vi "07_1.vi"() -> ()   [LabVIEW 2018]
uses:
  <userlib>/_OpenG.lib/array/array.llb/Remove Duplicates from 1D Array (String)__ogtk.vi
panel:
  out "Contained by Number":i32
  out "Contained by":string[](array[string])
  in  "Input":string="light chartreuse bags contain 1 mirrored yellow bag, 2 vibrant violet bags.\ndotted silver bags contain 2 dotted orange bags, 3 bright fuchsia bags, 5 bright tomato bags, 3 faded turquoise bags.\nplaid indigo bags contain 1 pale violet bag, 4 mirrored violet bags.\nfaded turquoise bags contain 5 faded lavender bags.\nstriped yellow bags contain 5 vibrant black bags, 1 mirrored gold bag.\ndull tan bags contain 1 vibrant aqua bag.\nstriped brown bags contain 1 vibrant orange bag, 1 posh bronze bag, 4 dim purple bags.\nbright teal bags contain 3 muted cyan bags, 2 drab white bags, 1 drab gray bag.\nwavy tan bags contain 4 wavy tomato bags, 1 dim tan bag.\nlight lavender bags contain 1 dotted black bag, 1 wavy maroon bag, 5 pale white bags, 1 clear tan bag.\ndull orange bags contain 5 bright brown bags, 1 muted gold bag, 4 vibrant black bags, 4 posh bronze bags.\nposh cyan bags contain 2 mirrored tomato bags, 5 light salmon bags, 1 faded brown bag, 4 vibrant red bags.\ndark lavender bags contain 2 faded purple bags.\ndark white bags contain 5 muted green bags.\nstriped olive bags contain 1 muted chartreuse bag.\nbright crimson bags contain 3 drab salmon bags, 1 faded plum bag, 4 shiny brown bags, 5 pale orange bags.\ndark tomato bags contain 5 dim aqua bags.\nlight olive bags contain 2 drab blue bags, 1 plaid purple bag.\nmuted gray bags contain 1 mirrored plum bag.\nbright salmon bags contain 3 striped plum bags, 1 dull silver bag, 4 striped indigo bags, 4 striped cyan bags.\nwavy gold bags contain 3 drab tomato bags, 5 pale gold bags, 1 plaid tan bag, 5 vibrant gold bags.\nmuted fuchsia bags contain 3 vibrant plum bags, 1 clear chartreuse bag, 1 pale white bag.\nlight purple bags contain 5 vibrant olive bags, 4 bright maroon bags, 3 posh tomato bags.\nvibrant gray bags contain 5 shiny silver bags.\nvibrant beige bags contain 2 pale crimson bags, 5 pale olive bags, 4 posh yellow bags, 3 dotted orange bags.\ndrab beige bags contain 3 faded gold bags, 5 mirrored fuchsia bags.\nlight white bags contain 1 vibrant fuchsia bag, 3 posh tomato bags, 4 muted chartreuse bags.\nposh lavender bags contain 3 dim fuchsia bags, 2 light violet bags, 3 wavy aqua bags, 5 vibrant lime bags.\nvibrant fuchsia bags contain 2 wavy tomato bags, 3 plaid purple bags.\nbright fuchsia bags contain 1 faded tomato bag, 4 bright salmon bags, 2 bright red bags.\ndim bronze bags contain 5 drab blue bags.\nwavy brown bags contain 3 dotted crimson bags.\nstriped plum bags contain 1 bright tomato bag.\nposh coral bags contain 1 mirrored gray bag, 1 posh silver bag.\nwavy teal bags contain 5 dark bronze bags.\nposh crimson bags contain 3 bright tomato bags, 3 wavy violet bags, 1 striped olive bag.\ndark beige bags contain 2 drab turquoise bags.\ndull green bags contain 2 vibrant purple bags, 5 dark red bags.\nwavy violet bags contain 5 faded lavender bags, 2 faded turquoise bags, 4 shiny brown bags.\nwavy crimson bags contain 3 muted lavender bags.\nlight maroon bags contain 1 bright magenta bag, 5 dim yellow bags, 1 faded violet bag.\nmuted white bags contain 4 muted purple bags, 2 plaid gray bags, 2 vibrant maroon bags.\nstriped silver bags contain 4 shiny red bags, 5 vibrant coral bags.\nclear chartreuse bags contain 3 pale gold bags.\nposh silver bags contain 3 vibrant aqua bags, 5 muted coral bags, 4 drab crimson bags, 4 clear tan bags.\nplaid green bags contain 1 striped lavender bag, 2 dim fuchsia bags, 5 vibrant black bags.\nmuted turquoise bags contain 3 faded green bags, 1 striped silver bag.\nfaded blue bags contain 3 pale crimson bags.\ndull magenta bags contain 2 striped brown bags, 4 posh black bags, 4 dark teal bags.\ndotted white bags contain 3 dotted magenta bags, 2 bright lavender bags, 5 drab crimson bags, 5 drab silver bags.\nshiny orange bags contain 4 pale violet bags.\nvibrant blue bags contain 2 clear yellow bags, 1 muted beige bag.\ndull blue bags contain 3 pale violet bags, 3 dotted orange bags.\nbright olive bags contain 4 dotted teal bags, 3 dotted violet bags.\nfaded gray bags contain 3 bright maroon bags, 2 shiny crimson bags, 2 plaid lavender bags.\nclear tomato bags contain 1 vibrant white bag, 4 bright gold bags, 3 vibrant chartreuse bags, 1 posh violet bag.\nbright indigo bags contain 3 wavy gold bags, 1 vibrant indigo bag, 1 mirrored chartreuse bag.\nclear indigo bags contain 1 plaid gray bag, 3 faded gold bags, 2 clear beige bags.\ndotted crimson bags contain 2 pale gold bags, 2 vibrant salmon bags, 5 posh maroon bags.\ndrab red bags contain 3 vibrant chartreuse bags, 5 wavy beige bags, 2 pale olive bags, 2 clear white bags.\nclear black bags contain 3 faded chartreuse bags, 2 striped brown bags, 4 wavy crimson bags, 3 pale tomato bags.\nshiny bronze bags contain 4 dark tan bags.\nposh indigo bags contain 1 clear plum bag, 2 dotted red bags, 1 dull crimson bag, 4 dotted bronze bags.\ndark cyan bags contain 3 plaid tan bags, 5 dim bronze bags.\nshiny chartreuse bags contain 4 dark tomato bags, 2 striped salmon bags.\ndim brown bags contain 1 pale olive bag, 4 posh tomato bags.\nfaded green bags contain 2 drab violet bags, 5 vibrant gray bags.\ndull salmon bags contain 5 muted coral bags, 2 muted brown bags, 2 striped coral bags, 5 dark white bags.\nwavy white bags contain 5 muted lime bags, 5 striped purple bags.\ndim aqua bags contain 2 striped beige bags, 3 striped silver bags, 1 bright cyan bag, 5 clear blue bags.\ndim salmon bags contain 5 mirrored lime bags, 1 vibrant plum bag, 5 mirrored fuchsia bags, 1 shiny gold bag.\ndotted fuchsia bags contain 4 striped indigo bags, 4 wavy coral bags.\nfaded tan bags contain 5 dotted gold bags.\ndrab white bags contain 3 posh violet bags.\nmuted teal bags contain 4 dotted purple bags, 5 dark maroon bags, 3 dotted magenta bags, 1 pale beige bag.\ndark magenta bags contain 3 posh red bags.\nshiny cyan bags contain 3 dull red bags, 1 light coral bag.\nplaid blue bags contain 3 shiny gold bags, 3 dull salmon bags, 4 vibrant silver bags, 4 light salmon bags.\ndim orange bags contain 5 vibrant salmon bags, 2 dotted teal bags.\nvibrant bronze bags contain 5 striped blue bags, 2 clear magenta bags.\nfaded olive bags contain 2 muted beige bags, 3 wavy beige bags.\ndotted lime bags contain 2 mirrored tan bags.\ndark silver bags contain 5 vibrant plum bags, 4 shiny gold bags, 3 light crimson bags, 2 dark cyan bags.\nmirrored orange bags contain 5 shiny blue bags, 4 faded olive bags, 3 posh gold bags.\nclear magenta bags contain 4 pale olive bags.\nwavy blue bags contain 4 light gray bags.\npale maroon bags contain 1 dim aqua bag, 3 dotted fuchsia bags, 1 clear brown bag, 1 drab turquoise bag.\nmuted purple bags contain no other bags.\nvibrant plum bags contain 5 wavy beige bags.\nmirrored gray bags contain 3 dull plum bags, 5 pale blue bags.\nstriped lavender bags contain 3 wavy tomato bags, 1 striped tan bag, 5 posh silver bags.\ndark violet bags contain 1 muted olive bag, 3 drab crimson bags.\nbright tomato bags contain 4 pale violet bags.\nposh white bags contain 5 clear white bags, 2 striped plum bags, 1 drab crimson bag, 5 wavy beige bags.\nstriped bronze bags contain 3 shiny teal bags, 5 bright lavender bags, 5 dark beige bags.\nclear beige bags contain 2 mirrored magenta bags, 4 muted olive bags, 4 mirrored violet bags.\nstriped teal bags contain 5 mirrored cyan bags, 3 posh crimson bags, 4 vibrant tan bags.\nbright blue bags contain 2 faded indigo bags, 4 wavy green bags.\nstriped orange bags contain 4 vibrant coral bags, 5 faded lavender bags, 2 vibrant maroon bags, 2 plaid cyan bags.\ndim yellow bags contain 5 pale violet bags, 4 muted plum bags, 5 pale coral bags, 4 pale yellow bags.\ndark bronze bags contain 5 posh gray bags.\nwavy purple bags contain 5 faded tomato bags, 4 striped green bags, 1 striped tan bag, 5 dotted fuchsia bags.\nlight fuchsia bags contain 5 shiny lime bags, 1 dotted teal bag, 2 muted brown bags.\nmuted orange bags contain 3 striped chartreuse bags, 4 dim salmon bags, 2 pale indigo bags.\ndotted green bags contain 5 dotted maroon bags, 4 vibrant beige bags, 3 striped beige bags.\nwavy gray bags contain 2 mirrored fuchsia bags, 2 mirrored chartreuse bags, 3 mirrored blue bags.\ndotted yellow bags contain 4 light tomato bags, 3 dull indigo bags.\nlight aqua bags contain 2 shiny brown bags, 2 bright coral bags.\nmuted cyan bags contain 5 faded olive bags, 5 pale white bags, 4 plaid tan bags.\npale tan bags contain 4 bright cyan bags.\nvibrant magenta bags contain 3 light magenta bags.\nlight turquoise bags contain 3 dim bronze bags, 3 faded olive bags, 1 light orange bag, 2 shiny green bags.\nlight bronze bags contain 2 vibrant black bags, 2 clear indigo bags.\nvibrant purple bags contain 3 bright red bags, 3 vibrant violet bags.\nvibrant red bags contain 4 mirrored fuchsia bags, 1 drab tomato bag.\nmirrored crimson bags contain 1 posh purple bag, 3 dotted magenta bags.\nwavy olive bags contain 3 dark fuchsia bags.\npale beige bags contain 5 striped coral bags, 1 shiny violet bag.\nposh teal bags contain 5 dull violet bags, 2 drab gold bags, 5 muted chartreuse bags, 1 drab turquoise bag.\nfaded tomato bags contain 5 mirrored salmon bags, 3 wavy coral bags.\nmuted salmon bags contain 4 vibrant gray bags.\ndim lavender bags contain 4 clear lavender bags, 5 dotted coral bags.\nshiny yellow bags contain 3 dim purple bags.\nlight tan bags contain 5 vibrant plum bags, 3 dim tomato bags.\nshiny violet bags contain 1 mirrored salmon bag.\ndrab black bags contain 2 dark coral bags, 1 muted beige bag, 5 plaid orange bags, 1 dark tan bag.\nwavy bronze bags contain 3 wavy lime bags, 3 striped white bags, 1 drab gray bag, 1 light orange bag.\nbright green bags contain 1 vibrant gold bag, 2 vibrant tomato bags, 2 dim teal bags.\nstriped gold bags contain 5 striped purple bags, 1 faded purple bag, 2 dark beige bags, 1 mirrored silver bag.\nwavy green bags contain 4 mirrored tan bags, 3 muted cyan bags, 4 plaid turquoise bags, 4 drab gray bags.\nstriped salmon bags contain 3 light yellow bags.\nbright orange bags contain 2 shiny orange bags.\nmirrored white bags contain 1 clear fuchsia bag.\nstriped coral bags contain no other bags.\nlight magenta bags contain 4 faded gold bags, 1 drab lime bag.\ndull tomato bags contain 4 pale indigo bags, 4 pale white bags, 5 wavy silver bags, 3 faded indigo bags.\nlight black bags contain 5 dark lavender bags, 3 light blue bags, 3 dull turquoise bags.\nposh fuchsia bags contain 1 wavy gold bag, 1 vibrant plum bag, 3 posh white bags.\nshiny indigo bags contain 3 posh plum bags, 2 pale lime bags, 5 muted blue bags, 4 clear tan bags.\nmirrored blue bags contain 3 dark indigo bags, 1 vibrant coral bag, 4 mirrored salmon bags.\npale tomato bags contain 3 plaid purple bags, 1 wavy violet bag.\ndull silver bags contain 4 striped beige bags, 2 shiny lime bags, 1 muted olive bag, 5 dull blue bags.\nmirrored silver bags contain 2 wavy coral bags, 3 dark lavender bags, 3 dull violet bags.\ndrab turquoise bags contain 2 dim purple bags, 5 clear white bags, 4 dull brown bags.\ndrab violet bags contain 1 pale white bag, 1 bright cyan bag.\npale indigo bags contain 4 striped blue bags, 1 plaid turquoise bag, 4 striped beige bags.\nshiny fuchsia bags contain 1 striped olive bag, 1 vibrant orange bag, 2 striped indigo bags, 4 vibrant lime bags.\nbright maroon bags contain 3 clear chartreuse bags.\nshiny tomato bags contain 5 pale gold bags, 5 plaid gold bags, 2 dark white bags.\ndotted olive bags contain 4 vibrant silver bags, 1 posh crimson bag.\ndrab teal bags contain 1 faded indigo bag.\nmuted plum bags contain 5 mirrored gray bags, 1 wavy maroon bag, 1 mirrored tomato bag, 3 drab crimson bags.\nmuted violet bags contain 5 drab crimson bags.\ndark brown bags contain 1 shiny violet bag, 5 bright coral bags, 4 vibrant plum bags, 3 plaid silver bags.\nposh purple bags contain 3 dull silver bags, 2 posh salmon bags, 5 dull chartreuse bags.\nlight yellow bags contain 5 striped olive bags, 2 mirrored tomato bags, 2 wavy plum bags.\nbright silver bags contain 4 pale bronze bags, 2 drab turquoise bags, 2 striped coral bags.\ndotted indigo bags contain 2 mirrored brown bags, 5 dim teal bags.\nbright lavender bags contain 3 dark indigo bags, 4 wavy brown bags, 3 dotted tomato bags, 5 plaid beige bags.\ndrab purple bags contain 5 mirrored bronze bags.\nclear olive bags contain 3 wavy red bags, 4 muted bronze bags, 2 dotted chartreuse bags.\nmirrored coral bags contain 4 shiny salmon bags, 1 light orange bag, 4 faded yellow bags, 5 shiny maroon bags.\nclear fuchsia bags contain 4 pale blue bags, 2 light lavender bags, 4 clear blue bags, 2 posh maroon bags.\ndrab fuchsia bags contain 4 drab bronze bags, 2 shiny bronze bags.\npale blue bags contain 2 dim purple bags, 3 plaid purple bags, 4 vibrant coral bags.\nclear violet bags contain 1 muted chartreuse bag.\nclear brown bags contain 3 faded chartreuse bags, 5 dotted plum bags, 2 mirrored plum bags, 4 plaid red bags.\nmuted maroon bags contain 1 muted chartreuse bag, 4 striped silver bags, 1 posh yellow bag, 4 dark indigo bags.\ndim olive bags contain 5 clear beige bags, 5 pale blue bags.\nbright violet bags contain 3 shiny salmon bags, 2 dull teal bags, 4 shiny blue bags, 2 posh teal bags.\ndrab green bags contain 5 wavy aqua bags, 5 dark lavender bags, 1 dull tan bag.\ndim turquoise bags contain 2 dark brown bags, 3 dotted crimson bags, 3 dull salmon bags.\nvibrant teal bags contain 2 dotted coral bags, 5 dim white bags.\nposh maroon bags contain 3 muted purple bags, 2 bright tomato bags.\nfaded aqua bags contain 4 posh white bags, 2 mirrored violet bags.\nvibrant violet bags contain 2 vibrant crimson bags, 2 drab crimson bags.\ndotted salmon bags contain 3 faded violet bags, 4 clear beige bags, 2 bright coral bags.\ndull chartreuse bags contain 1 dotted fuchsia bag, 5 posh black bags, 4 bright green bags.\nvibrant orange bags contain 1 shiny green bag, 5 dull blue bags.\nmirrored indigo bags contain 2 dull beige bags.\ndrab lavender bags contain 3 striped lime bags.\nbright gold bags contain 5 posh silver bags.\ndull fuchsia bags contain 2 striped tomato bags.\nlight lime bags contain 3 striped orange bags.\nwavy magenta bags contain 3 clear fuchsia bags, 4 muted brown bags, 3 plaid lavender bags, 4 clear green bags.\nfaded beige bags contain 2 mirrored plum bags, 2 light blue bags, 4 dim purple bags, 5 plaid violet bags.\ndark plum bags contain 2 shiny red bags, 5 shiny blue bags, 2 striped blue bags, 4 drab gray bags.\nwavy turquoise bags contain 1 dim turquoise bag, 5 striped lavender bags, 3 drab aqua bags.\nshiny white bags contain 4 shiny violet bags, 1 muted bronze bag, 3 clear tomato bags.\nplaid yellow bags contain 4 vibrant indigo bags, 2 light gray bags.\ndim crimson bags contain 5 dim brown bags, 3 dim white bags, 1 vibrant silver bag, 3 drab teal bags.\ndim tomato bags contain 4 dull silver bags, 5 light gray bags.\nwavy cyan bags contain 5 dark chartreuse bags, 1 dark maroon bag, 4 mirrored brown bags, 5 dotted fuchsia bags.\ndim green bags contain 5 striped lime bags, 4 bright gold bags, 2 vibrant violet bags, 2 muted beige bags.\nstriped maroon bags contain 1 mirrored plum bag, 1 drab lavender bag, 5 posh teal bags.\ndotted gray bags contain 3 vibrant white bags, 1 pale violet bag.\ndotted beige bags contain 2 drab aqua bags.\nclear crimson bags contain 2 dim white bags, 2 faded magenta bags, 1 dim tomato bag.\npale olive bags contain 2 posh tomato bags.\nposh orange bags contain 3 muted cyan bags, 4 faded turquoise bags.\nposh yellow bags contain 2 dotted orange bags, 2 striped crimson bags.\nstriped black bags contain 5 dark black bags, 2 faded magenta bags, 3 pale lavender bags.\nfaded orange bags contain 4 bright bronze bags.\npale turquoise bags contain 1 posh maroon bag, 4 faded violet bags, 2 faded lavender bags, 1 vibrant lime bag.\nclear gray bags contain 4 posh gray bags, 4 shiny silver bags, 3 vibrant purple bags, 3 faded lavender bags.\nshiny olive bags contain 4 vibrant lime bags, 5 faded coral bags.\nvibrant maroon bags contain 5 light gray bags.\ndrab silver bags contain 3 vibrant salmon bags, 5 clear tan bags, 2 light white bags.\nposh turquoise bags contain 5 plaid green bags, 2 light bronze bags, 4 shiny turquoise bags, 5 clear gray bags.\nmirrored cyan bags contain 3 clear white bags.\nshiny silver bags contain 4 vibrant coral bags.\nclear plum bags contain 5 muted lavender bags, 5 striped coral bags.\ndark crimson bags contain 4 posh violet bags.\nmuted red bags contain 1 dim maroon bag, 1 bright fuchsia bag, 3 dotted green bags, 3 striped gold bags.\nclear lime bags contain 3 plaid cyan bags, 4 dim gray bags, 1 muted violet bag.\nfaded purple bags contain 3 muted beige bags, 1 posh white bag, 5 drab turquoise bags.\nmirrored yellow bags contain 2 striped tan bags.\ndim gray bags contain 3 bright green bags, 2 muted black bags, 5 mirrored maroon bags, 3 mirrored violet bags.\nmirrored tomato bags contain 5 muted olive bags, 2 mirrored lime bags.\nfaded coral bags contain 3 bright brown bags, 4 vibrant purple bags, 3 posh coral bags.\nwavy fuchsia bags contain 4 dim salmon bags, 4 vibrant violet bags, 5 muted beige bags, 2 dotted black bags.\nlight plum bags contain 1 wavy black bag.\ndark tan bags contain 5 wavy green bags, 4 faded turquoise bags, 2 dark bronze bags, 3 light violet bags.\nwavy beige bags contain no other bags.\ndotted aqua bags contain 1 mirrored turquoise bag, 4 clear blue bags, 1 dotted teal bag, 3 bright bronze bags.\nclear tan bags contain 3 clear gold bags, 3 plaid purple bags, 1 striped indigo bag, 5 bright tomato bags.\ndark red bags contain 3 vibrant maroon bags, 3 vibrant fuchsia bags, 4 pale lavender bags, 4 dim purple bags.\ndim violet bags contain 1 drab tomato bag, 2 vibrant white bags, 3 faded lavender bags.\ndull gray bags contain 3 vibrant black bags.\nmirrored aqua bags contain 4 clear fuchsia bags, 1 muted chartreuse bag.\npale violet bags contain no other bags.\nfaded silver bags contain 1 mirrored lime bag, 5 muted beige bags, 3 mirrored black bags, 1 clear gold bag.\nposh tomato bags contain 3 dim purple bags, 1 vibrant maroon bag.\nmirrored bronze bags contain 3 mirrored gold bags, 4 faded purple bags, 1 plaid cyan bag, 5 faded gold bags.\nlight red bags contain 3 muted black bags.\nwavy salmon bags contain 1 light white bag, 1 clear white bag, 4 dark maroon bags.\nposh lime bags contain 2 drab gold bags.\nwavy chartreuse bags contain 4 muted teal bags, 3 plaid salmon bags.\ndotted tomato bags contain 2 striped white bags, 4 dark lavender bags.\nvibrant crimson bags contain no other bags.\nposh violet bags contain 1 shiny lavender bag, 2 striped coral bags, 2 mirrored tan bags.\nshiny lime bags contain 5 mirrored lime bags, 1 drab blue bag.\ndotted magenta bags contain 5 bright salmon bags.\npale white bags contain 1 faded olive bag, 5 vibrant tomato bags.\nmuted lime bags contain 3 muted aqua bags.\ndotted lavender bags contain 2 dim chartreuse bags, 2 vibrant olive bags.\nfaded crimson bags contain 4 bright plum bags, 5 dotted cyan bags.\ndrab tan bags contain 1 dim orange bag, 2 light teal bags, 2 light indigo bags.\npale black bags contain 2 posh silver bags.\ndark orange bags contain 3 muted black bags, 2 pale violet bags, 4 faded cyan bags.\nmirrored violet bags contain 1 faded olive bag, 3 vibrant crimson bags.\nposh plum bags contain 3 vibrant maroon bags.\nclear turquoise bags contain 1 dim purple bag.\nplaid gray bags contain 1 dotted crimson bag.\npale salmon bags contain 4 vibrant aqua bags, 2 wavy blue bags, 5 striped violet bags.\npale gold bags contain 1 striped coral bag.\nbright plum bags contain 5 faded aqua bags.\npale red bags contain 5 dotted silver bags, 3 clear chartreuse bags, 4 vibrant salmon bags.\nstriped tan bags contain 1 drab crimson bag.\nmirrored red bags contain 3 striped gold bags, 1 mirrored gray bag.\nbright turquoise bags contain 2 plaid blue bags, 4 clear tomato bags, 1 drab yellow bag, 5 vibrant black bags.\ndark maroon bags contain 5 shiny magenta bags, 5 dotted fuchsia bags, 5 dull brown bags, 5 posh violet bags.\nplaid chartreuse bags contain 5 drab gold bags, 1 vibrant white bag, 3 muted coral bags, 2 clear plum bags.\nposh black bags contain 5 shiny brown bags, 5 posh white bags, 4 dim gray bags.\ndotted teal bags contain 1 plaid bronze bag, 2 light violet bags, 1 muted beige bag.\nplaid lime bags contain 4 mirrored black bags, 4 muted plum bags, 2 shiny maroon bags, 5 dim beige bags.\ndim teal bags contain 2 muted coral bags.\nvibrant aqua bags contain no other bags.\ndotted turquoise bags contain 3 posh violet bags.\nvibrant lime bags contain 5 dark bronze bags, 3 vibrant maroon bags, 5 mirrored cyan bags.\nshiny gray bags contain 3 muted coral bags, 2 bright coral bags.\nclear white bags contain 1 dim purple bag.\nshiny salmon bags contain 5 dull tan bags, 1 posh violet bag, 4 mirrored magenta bags, 5 plaid tan bags.\ndark gold bags contain 5 mirrored gray bags, 4 vibrant coral bags.\ndrab salmon bags contain 1 dull indigo bag.\nfaded salmon bags contain 2 bright blue bags.\nvibrant salmon bags contain 4 muted purple bags, 4 striped plum bags.\ndull red bags contain 2 pale white bags.\nmuted yellow bags contain 3 pale beige bags, 2 dim indigo bags.\nbright beige bags contain 1 muted lavender bag, 1 dotted silver bag, 1 shiny bronze bag.\ndull gold bags contain 4 posh gold bags.\nstriped crimson bags contain 5 dull blue bags, 4 bright gold bags, 2 shiny lavender bags.\ndrab maroon bags contain 1 wavy fuchsia bag.\nwavy plum bags contain 4 posh tan bags, 1 muted maroon bag.\nbright black bags contain 4 dark white bags, 5 dull maroon bags.\nplaid aqua bags contain 3 wavy gray bags, 4 shiny blue bags.\nwavy silver bags contain 1 bright tomato bag.\nclear orange bags contain 1 dark brown bag, 3 wavy bronze bags, 5 bright tomato bags, 2 faded olive bags.\nshiny lavender bags contain 4 dim purple bags.\ndull crimson bags contain 5 bright plum bags, 1 pale yellow bag.\nvibrant brown bags contain 2 dull tan bags, 1 pale yellow bag, 5 striped orange bags.\nstriped white bags contain 5 pale orange bags.\nlight blue bags contain 1 vibrant red bag, 3 bright cyan bags, 5 vibrant brown bags, 5 dim beige bags.\ndark green bags contain 4 dotted black bags.\nplaid black bags contain 5 dotted chartreuse bags, 1 wavy yellow bag, 4 faded cyan bags, 5 posh orange bags.\nshiny turquoise bags contain 5 vibrant tan bags, 1 vibrant salmon bag, 1 muted olive bag.\nclear silver bags contain 3 drab crimson bags, 3 bright magenta bags, 5 shiny blue bags, 4 drab lavender bags.\nmuted chartreuse bags contain 2 mirrored tan bags.\nmirrored brown bags contain 5 clear yellow bags, 3 clear violet bags, 1 wavy plum bag.\ndull white bags contain 5 shiny blue bags, 2 plaid tan bags, 3 vibrant silver bags, 4 pale orange bags.\nclear lavender bags contain 2 posh bronze bags.\nlight gold bags contain 3 striped cyan bags, 5 dark lime bags.\nplaid coral bags contain 1 posh salmon bag, 1 striped purple bag, 4 bright blue bags.\nfaded magenta bags contain 1 posh yellow bag, 2 bright plum bags.\nfaded maroon bags contain 2 plaid gray bags.\nclear green bags contain 5 vibrant silver bags, 4 shiny gold bags.\nmirrored tan bags contain 2 plaid purple bags, 4 dim purple bags, 5 vibrant crimson bags.\nstriped red bags contain 2 clear salmon bags.\ndull aqua bags contain 1 plaid red bag, 3 vibrant aqua bags.\nbright coral bags contain 4 muted fuchsia bags, 4 wavy beige bags.\nwavy black bags contain 3 drab crimson bags, 3 vibrant white bags, 4 vibrant aqua bags.\ndim white bags contain 1 dull olive bag, 5 vibrant white bags.\nstriped turquoise bags contain 2 drab turquoise bags.\nshiny gold bags contain 2 mirrored blue bags, 1 muted brown bag, 3 dim purple bags.\nbright gray bags contain 1 faded cyan bag, 3 dark plum bags, 1 light violet bag.\nmirrored olive bags contain 5 vibrant gray bags, 1 plaid blue bag, 5 clear black bags, 2 dotted black bags.\nposh red bags contain 5 muted olive bags, 2 dotted coral bags, 1 striped crimson bag.\nclear teal bags contain 4 bright gold bags, 5 striped gray bags, 2 mirrored lime bags, 4 wavy indigo bags.\nfaded lime bags contain 4 plaid beige bags.\ndull yellow bags contain 1 clear indigo bag, 1 drab beige bag, 2 plaid bronze bags.\nmuted beige bags contain no other bags.\nwavy orange bags contain 3 shiny lime bags, 4 striped gold bags.\ndrab brown bags contain 1 bright red bag, 1 posh yellow bag, 3 dotted gray bags, 2 plaid green bags.\nmuted olive bags contain 4 posh maroon bags, 4 bright maroon bags, 3 faded olive bags.\ndotted cyan bags contain 5 dotted purple bags, 5 pale olive bags, 5 dull plum bags.\nvibrant olive bags contain 2 light violet bags, 2 dim violet bags, 4 mirrored black bags.\npale lime bags contain 4 dark purple bags, 1 shiny chartreuse bag.\ndull purple bags contain 1 faded blue bag, 4 dull violet bags, 2 dim bronze bags, 2 vibrant crimson bags.\ndotted red bags contain 4 bright magenta bags, 1 mirrored cyan bag, 1 wavy green bag, 4 dotted cyan bags.\nvibrant silver bags contain 4 faded purple bags, 3 shiny yellow bags, 4 mirrored tan bags.\ndark fuchsia bags contain 3 dark cyan bags.\nmuted crimson bags contain 3 bright tomato bags, 4 dark gold bags.\ndark coral bags contain 3 faded magenta bags.\ndull teal bags contain 3 drab turquoise bags, 5 dim salmon bags, 2 striped coral bags.\nlight brown bags contain 5 bright tomato bags, 4 mirrored salmon bags, 2 vibrant violet bags, 5 dark bronze bags.\nbright brown bags contain 3 muted purple bags, 2 vibrant yellow bags, 3 pale fuchsia bags, 3 posh violet bags.\nfaded bronze bags contain 2 bright bronze bags, 2 dim tomato bags, 3 mirrored beige bags.\ndim indigo bags contain 2 vibrant gold bags.\ndrab cyan bags contain 5 muted orange bags, 4 dotted orange bags, 3 striped tan bags, 5 dull turquoise bags.\nmirrored plum bags contain 1 dotted black bag, 2 faded silver bags, 1 plaid red bag.\ndull maroon bags contain 5 dark violet bags, 2 bright brown bags, 4 clear blue bags.\nlight silver bags contain 3 bright blue bags, 1 muted brown bag.\ndim blue bags contain 5 dim purple bags, 5 pale orange bags.\nclear blue bags contain 2 plaid tan bags, 3 muted chartreuse bags, 2 faded lavender bags.\nmirrored salmon bags contain 2 striped coral bags, 2 plaid purple bags.\nfaded violet bags contain 3 clear gold bags, 2 posh white bags.\nlight beige bags contain 5 vibrant tan bags, 4 muted lavender bags, 3 plaid bronze bags.\nshiny black bags contain 3 vibrant violet bags, 1 wavy brown bag.\ndotted plum bags contain 4 faded yellow bags, 5 light lavender bags.\nvibrant chartreuse bags contain 1 mirrored fuchsia bag.\nstriped green bags contain 2 wavy lime bags, 5 mirrored turquoise bags, 2 muted aqua bags, 3 wavy gold bags.\nplaid plum bags contain 5 plaid tan bags, 2 pale gold bags, 5 mirrored salmon bags.\ndark chartreuse bags contain 1 bright orange bag, 5 bright lavender bags, 2 light black bags.\nmuted indigo bags contain 2 posh fuchsia bags.\nposh tan bags contain 3 dull silver bags, 2 clear tan bags, 4 drab beige bags.\nshiny brown bags contain 5 shiny gold bags.\npale orange bags contain 2 striped gray bags, 5 clear beige bags.\npale lavender bags contain 1 shiny lime bag, 1 bright cyan bag.\npale bronze bags contain 2 faded blue bags, 4 pale yellow bags, 5 shiny red bags.\nmuted bronze bags contain 3 light beige bags, 4 muted fuchsia bags, 5 striped chartreuse bags.\nlight crimson bags contain 2 faded coral bags.\ndrab coral bags contain 4 faded black bags, 4 drab white bags, 5 wavy maroon bags, 4 muted violet bags.\nvibrant lavender bags contain 2 striped crimson bags.\nposh magenta bags contain 1 bright chartreuse bag, 3 drab white bags, 4 dull violet bags.\ndim maroon bags contain 1 drab lime bag, 4 faded aqua bags, 5 dark lavender bags.\nclear purple bags contain 1 pale lavender bag.\ndim magenta bags contain 3 dull violet bags, 4 pale red bags.\nplaid red bags contain 5 clear indigo bags.\nlight gray bags contain 2 dark white bags, 5 posh green bags, 1 wavy silver bag.\nplaid beige bags contain 2 dotted brown bags, 2 clear white bags.\nfaded gold bags contain 2 clear white bags, 1 muted purple bag, 1 striped plum bag.\ndrab yellow bags contain 3 striped lime bags, 5 muted fuchsia bags, 1 wavy black bag, 3 pale white bags.\ndark indigo bags contain 4 striped indigo bags, 4 mirrored violet bags, 3 muted brown bags.\nmuted black bags contain 1 plaid tan bag, 2 bright tomato bags.\nshiny beige bags contain 5 dark bronze bags.\nbright cyan bags contain 2 dark lavender bags, 5 striped plum bags, 3 mirrored tan bags, 5 plaid teal bags.\ndotted gold bags contain 2 pale gold bags, 1 drab silver bag.\nwavy tomato bags contain 4 dotted crimson bags, 4 mirrored lime bags, 2 dim indigo bags.\nmuted aqua bags contain 3 muted beige bags.\nplaid white bags contain 2 bright green bags, 3 mirrored blue bags, 3 dull maroon bags, 2 dotted chartreuse bags.\nplaid teal bags contain 1 plaid tan bag, 3 wavy beige bags.\nlight salmon bags contain 5 faded turquoise bags, 5 muted green bags, 2 plaid bronze bags, 3 plaid indigo bags.\ndark aqua bags contain 2 wavy plum bags, 2 dotted red bags, 2 light red bags.\npale aqua bags contain 4 light aqua bags, 4 clear cyan bags, 5 dull tan bags, 5 bright olive bags.\nposh green bags contain 5 pale blue bags.\nfaded chartreuse bags contain 2 shiny red bags.\npale purple bags contain 2 mirrored cyan bags.\nstriped magenta bags contain 1 muted aqua bag, 1 plaid turquoise bag, 5 dim purple bags, 3 wavy red bags.\nplaid crimson bags contain 5 muted brown bags, 5 mirrored tomato bags.\nplaid orange bags contain 1 dotted salmon bag, 2 pale aqua bags, 4 shiny tomato bags, 1 dull salmon bag.\nfaded red bags contain 1 clear tan bag.\nplaid fuchsia bags contain 1 dark black bag, 1 dotted teal bag, 2 dark aqua bags, 2 dull bronze bags.\npale crimson bags contain 5 dull brown bags, 3 vibrant coral bags.\nmuted lavender bags contain 2 posh silver bags, 1 plaid cyan bag.\ndull violet bags contain 5 posh coral bags, 5 shiny red bags, 5 drab gold bags, 4 posh white bags.\ndull coral bags contain 5 bright lime bags.\nposh gold bags contain 1 vibrant violet bag, 1 muted lavender bag.\ndrab lime bags contain 4 shiny salmon bags, 1 plaid plum bag, 1 wavy tomato bag, 1 wavy red bag.\nplaid tan bags contain 3 muted purple bags.\nposh chartreuse bags contain 5 clear white bags, 2 dotted violet bags, 5 light teal bags, 5 vibrant gold bags.\nfaded yellow bags contain 1 muted coral bag, 3 shiny yellow bags, 4 shiny lime bags.\nvibrant cyan bags contain 3 muted purple bags, 4 pale tomato bags, 4 vibrant beige bags, 2 muted black bags.\nplaid tomato bags contain 3 faded fuchsia bags.\ndotted maroon bags contain 4 dull tan bags, 4 plaid cyan bags, 5 bright gold bags, 4 drab blue bags.\ndrab gray bags contain 4 faded olive bags, 3 vibrant crimson bags.\nwavy maroon bags contain 1 wavy red bag, 4 posh white bags, 4 wavy tomato bags.\ndull lavender bags contain 2 dim salmon bags, 3 dotted aqua bags, 2 dim turquoise bags, 4 muted gold bags.\ndim chartreuse bags contain 4 muted yellow bags, 1 muted violet bag, 2 shiny orange bags, 4 drab salmon bags.\nbright red bags contain 1 dull red bag, 1 muted fuchsia bag.\nclear yellow bags contain 2 dim violet bags, 5 dim tomato bags, 4 pale indigo bags.\nwavy aqua bags contain 5 shiny red bags, 1 pale gold bag, 2 mirrored blue bags, 4 dull violet bags.\nbright lime bags contain 5 posh tomato bags, 2 faded fuchsia bags, 4 posh yellow bags, 5 dull brown bags.\nbright chartreuse bags contain 2 posh fuchsia bags, 1 posh yellow bag, 3 dotted chartreuse bags.\nmirrored magenta bags contain 1 shiny teal bag, 1 mirrored maroon bag, 3 drab turquoise bags.\npale yellow bags contain 3 plaid purple bags, 2 vibrant black bags.\ndark teal bags contain 4 clear salmon bags, 3 mirrored blue bags, 3 pale blue bags.\nclear coral bags contain 2 dark indigo bags, 5 dark plum bags, 5 plaid beige bags.\nmuted brown bags contain no other bags.\ndotted purple bags contain 1 posh bronze bag, 1 vibrant chartreuse bag, 5 striped indigo bags.\nplaid violet bags contain 2 posh white bags.\ndull turquoise bags contain 1 drab red bag, 5 muted aqua bags, 4 drab violet bags, 2 muted purple bags.\nlight coral bags contain 3 posh bronze bags, 5 vibrant silver bags.\nstriped lime bags contain 5 muted olive bags.\npale cyan bags contain 2 mirrored tomato bags, 3 dull red bags, 4 striped indigo bags, 2 dark maroon bags.\nmuted tomato bags contain 2 posh tomato bags, 3 dim teal bags, 4 drab indigo bags.\nshiny coral bags contain 4 mirrored beige bags, 1 muted magenta bag, 2 light green bags, 3 mirrored olive bags.\nvibrant black bags contain 2 dotted black bags, 4 dull red bags, 2 light lavender bags.\nvibrant green bags contain 5 mirrored bronze bags, 5 dotted teal bags, 5 plaid tomato bags, 2 muted purple bags.\nclear aqua bags contain 2 plaid teal bags, 3 posh tomato bags, 3 light bronze bags, 3 posh teal bags.\ndotted brown bags contain 5 pale white bags, 2 dim indigo bags, 1 shiny yellow bag, 3 plaid gray bags.\nstriped beige bags contain 3 striped indigo bags, 4 faded lavender bags, 1 drab crimson bag, 1 vibrant tomato bag.\nplaid cyan bags contain 4 shiny gold bags, 1 wavy beige bag.\nmirrored gold bags contain 3 vibrant coral bags.\nplaid turquoise bags contain 5 striped coral bags.\npale magenta bags contain 1 drab tomato bag, 4 dark chartreuse bags, 4 striped tan bags, 5 vibrant white bags.\npale green bags contain 4 shiny tan bags.\nfaded indigo bags contain 3 bright plum bags, 3 posh teal bags.\ndim red bags contain 2 striped silver bags, 4 dim blue bags.\nbright tan bags contain 1 vibrant cyan bag, 5 mirrored magenta bags.\ndotted violet bags contain 1 bright bronze bag, 4 dotted silver bags, 1 drab silver bag, 4 plaid indigo bags.\ndim black bags contain 1 dark magenta bag, 4 vibrant tan bags, 5 light magenta bags.\nbright aqua bags contain 2 muted gold bags, 3 dotted gray bags.\nplaid salmon bags contain 2 vibrant gold bags, 2 bright maroon bags, 2 shiny lime bags, 2 mirrored salmon bags.\ndrab chartreuse bags contain 3 shiny crimson bags.\nshiny magenta bags contain 2 striped plum bags.\ndotted blue bags contain 2 muted salmon bags.\nbright white bags contain 2 pale olive bags, 2 dotted black bags.\nclear red bags contain 2 bright chartreuse bags, 5 striped magenta bags.\nmirrored chartreuse bags contain 2 vibrant crimson bags, 2 drab blue bags.\nstriped fuchsia bags contain 2 muted salmon bags, 2 posh bronze bags.\nposh blue bags contain 2 faded bronze bags, 4 striped purple bags.\nmirrored fuchsia bags contain 5 mirrored tan bags, 4 muted coral bags.\nposh beige bags contain 5 drab violet bags.\nstriped violet bags contain 2 wavy plum bags, 1 pale crimson bag.\nvibrant turquoise bags contain 4 plaid gray bags.\ndotted bronze bags contain 2 drab maroon bags, 4 posh plum bags, 2 dotted brown bags, 5 mirrored cyan bags.\ndim cyan bags contain 2 pale orange bags, 2 posh white bags, 3 plaid salmon bags.\nvibrant gold bags contain 1 bright coral bag, 2 mirrored black bags.\nposh bronze bags contain 3 bright green bags, 5 faded turquoise bags, 5 plaid plum bags, 3 dull tan bags.\npale chartreuse bags contain 3 vibrant gray bags, 5 posh coral bags, 5 bright white bags, 4 faded white bags.\ndrab crimson bags contain 2 wavy beige bags, 3 striped coral bags, 1 dim purple bag, 3 pale gold bags.\nmirrored lime bags contain 5 striped coral bags, 2 wavy beige bags.\nshiny green bags contain 4 plaid silver bags, 2 dim teal bags, 2 dotted teal bags, 2 drab turquoise bags.\nlight tomato bags contain 4 dark gold bags.\nmirrored beige bags contain 5 posh gray bags, 5 dull olive bags, 3 drab crimson bags, 4 striped silver bags.\nvibrant indigo bags contain 2 pale brown bags, 2 vibrant tomato bags, 3 dim violet bags.\ndim plum bags contain 1 plaid aqua bag, 1 wavy plum bag, 1 wavy aqua bag.\nlight indigo bags contain 4 mirrored purple bags.\nfaded brown bags contain 2 dim gold bags.\ndim gold bags contain 4 dotted purple bags, 5 dotted black bags, 4 vibrant beige bags, 4 clear magenta bags.\nclear cyan bags contain 1 mirrored blue bag, 5 clear gray bags.\ndark yellow bags contain 3 dull violet bags, 3 dotted crimson bags, 1 dark bronze bag, 3 vibrant tomato bags.\nplaid silver bags contain 5 drab gray bags.\nvibrant yellow bags contain 5 plaid teal bags, 1 shiny silver bag, 1 mirrored black bag.\ndull olive bags contain 1 dark bronze bag, 5 wavy green bags, 2 muted cyan bags.\nplaid brown bags contain 3 drab indigo bags.\nfaded cyan bags contain 3 light lavender bags.\ndrab orange bags contain 5 plaid teal bags, 1 clear fuchsia bag.\nmuted tan bags contain 4 faded bronze bags, 4 vibrant green bags.\ndull cyan bags contain 5 striped maroon bags, 2 dim plum bags.\nwavy red bags contain 3 mirrored fuchsia bags, 5 vibrant salmon bags.\nwavy lime bags contain 5 faded lavender bags, 1 posh maroon bag.\ndotted tan bags contain 2 shiny teal bags, 2 plaid gray bags, 2 pale silver bags, 3 dim violet bags.\nclear salmon bags contain 4 striped white bags, 3 light coral bags, 1 mirrored white bag, 5 dotted silver bags.\ndark purple bags contain 1 shiny lime bag, 3 dull salmon bags.\ndim purple bags contain 5 wavy beige bags, 5 vibrant aqua bags, 5 muted purple bags.\nstriped gray bags contain 5 muted lavender bags, 1 clear blue bag.\nbright yellow bags contain 4 bright fuchsia bags, 3 drab brown bags, 5 shiny lime bags.\nlight teal bags contain 5 faded olive bags.\nwavy yellow bags contain 2 striped cyan bags, 5 dim indigo bags.\nvibrant tomato bags contain 2 shiny violet bags, 2 mirrored blue bags, 1 pale violet bag, 2 faded olive bags.\npale silver bags contain 2 dotted magenta bags, 2 mirrored salmon bags, 2 dim blue bags.\nmirrored lavender bags contain 3 pale teal bags, 2 posh gray bags.\nstriped chartreuse bags contain 3 plaid bronze bags.\ndotted chartreuse bags contain 1 pale white bag, 1 striped tan bag, 1 striped beige bag, 1 dull brown bag.\nmuted silver bags contain 2 shiny tan bags, 5 mirrored red bags, 3 drab brown bags.\nclear maroon bags contain 1 shiny gray bag, 4 posh purple bags, 5 pale silver bags.\nlight cyan bags contain 3 vibrant yellow bags.\nplaid magenta bags contain 3 bright olive bags, 2 faded violet bags, 1 bright salmon bag.\ndrab gold bags contain 1 dull blue bag, 5 mirrored gold bags, 3 striped cyan bags, 3 mirrored cyan bags.\nlight green bags contain 3 dotted brown bags.\ndim silver bags contain 2 pale cyan bags, 3 muted gold bags, 2 faded fuchsia bags.\nfaded black bags contain 5 dim orange bags, 2 shiny green bags, 2 faded cyan bags, 3 dull yellow bags.\nbright bronze bags contain 5 plaid indigo bags.\nlight orange bags contain 4 wavy beige bags, 5 mirrored blue bags, 5 faded turquoise bags.\ndark black bags contain 1 posh maroon bag, 1 faded turquoise bag, 2 drab violet bags, 4 mirrored white bags.\ndark gray bags contain 3 dotted coral bags, 3 plaid bronze bags.\nshiny aqua bags contain 1 muted coral bag.\nstriped aqua bags contain 2 posh bronze bags.\ndull plum bags contain 4 drab gray bags, 5 posh maroon bags.\nposh salmon bags contain 2 mirrored bronze bags, 5 plaid aqua bags.\nmuted blue bags contain 1 drab yellow bag.\ndim lime bags contain 4 plaid teal bags, 5 dotted orange bags, 5 wavy silver bags, 3 muted purple bags.\nstriped cyan bags contain 1 mirrored chartreuse bag.\ndull beige bags contain 3 drab red bags, 4 vibrant olive bags.\nwavy indigo bags contain 4 pale orange bags, 1 vibrant salmon bag, 5 wavy red bags, 2 plaid indigo bags.\ndrab tomato bags contain 3 clear gold bags.\nshiny crimson bags contain 2 vibrant lime bags, 5 shiny lavender bags, 3 dark purple bags, 3 light beige bags.\nbright magenta bags contain 4 striped gray bags, 5 dim cyan bags.\nplaid maroon bags contain 1 bright magenta bag, 2 dark olive bags.\nfaded white bags contain 2 faded turquoise bags.\npale plum bags contain 3 clear beige bags, 1 mirrored violet bag.\ndim fuchsia bags contain 1 posh maroon bag, 1 dull tan bag.\ndark olive bags contain 4 clear chartreuse bags, 5 light cyan bags, 5 striped magenta bags.\ndull lime bags contain 1 striped lavender bag, 1 shiny lavender bag, 2 faded cyan bags.\nfaded fuchsia bags contain 4 wavy aqua bags, 3 dark brown bags, 1 pale orange bag, 3 striped indigo bags.\nposh olive bags contain 3 drab maroon bags, 1 vibrant white bag, 2 wavy lime bags, 5 drab purple bags.\ndull black bags contain 4 posh tomato bags, 4 wavy aqua bags, 2 dull tomato bags, 2 clear orange bags.\nstriped blue bags contain 5 pale crimson bags, 5 clear chartreuse bags.\nshiny blue bags contain 1 plaid tan bag, 1 plaid silver bag.\ndrab bronze bags contain 5 faded fuchsia bags.\nposh aqua bags contain 3 dull turquoise bags, 5 dim olive bags.\nplaid lavender bags contain 5 mirrored red bags, 1 striped salmon bag, 2 mirrored turquoise bags, 4 dotted cyan bags.\nshiny purple bags contain 1 vibrant coral bag, 1 striped blue bag.\nmirrored purple bags contain 3 plaid teal bags.\nvibrant coral bags contain 1 striped coral bag, 4 pale gold bags.\ndrab blue bags contain 4 drab gray bags, 4 vibrant coral bags, 1 plaid teal bag.\nmirrored green bags contain 2 dull brown bags, 1 faded white bag.\ndim beige bags contain 3 clear blue bags, 1 shiny magenta bag.\nstriped tomato bags contain 4 vibrant silver bags, 2 bright yellow bags.\nclear bronze bags contain 5 striped coral bags, 3 wavy green bags, 1 bright violet bag.\nshiny teal bags contain 1 drab white bag.\nfaded lavender bags contain 5 dim teal bags, 2 faded olive bags, 2 dim purple bags, 2 pale gold bags.\nposh gray bags contain 2 mirrored tan bags.\npale brown bags contain 5 dull tan bags, 2 posh tomato bags.\nshiny plum bags contain 2 mirrored blue bags, 5 dark cyan bags, 2 dark teal bags.\nwavy lavender bags contain 1 wavy gold bag, 2 wavy maroon bags, 2 dark black bags.\nshiny tan bags contain 3 bright bronze bags, 1 posh fuchsia bag, 1 dark maroon bag, 4 wavy salmon bags.\ndim coral bags contain 3 faded indigo bags, 5 clear white bags.\nmirrored turquoise bags contain 4 vibrant coral bags, 4 pale gold bags, 1 clear blue bag.\nmuted coral bags contain no other bags.\ndrab plum bags contain 4 drab gray bags, 4 dotted green bags, 2 bright gray bags.\nmuted gold bags contain 3 shiny red bags, 5 light white bags, 3 mirrored maroon bags.\nlight violet bags contain 1 plaid tan bag, 2 plaid turquoise bags.\ndotted coral bags contain 4 dark crimson bags, 3 muted plum bags, 2 vibrant black bags, 4 drab gray bags.\npale fuchsia bags contain 3 dark brown bags.\ndark turquoise bags contain 3 plaid teal bags, 5 dull orange bags.\ndark blue bags contain 4 drab silver bags, 2 shiny brown bags.\nmuted green bags contain 1 mirrored violet bag, 3 posh silver bags, 2 bright coral bags, 4 clear chartreuse bags.\nposh brown bags contain 2 mirrored turquoise bags.\nvibrant tan bags contain 3 drab gray bags.\ndull indigo bags contain 1 dim tomato bag, 3 pale brown bags.\npale teal bags contain 3 light beige bags, 1 plaid indigo bag, 3 striped tan bags, 5 vibrant white bags.\nstriped purple bags contain 2 drab white bags.\npale coral bags contain 3 plaid teal bags.\nclear gold bags contain 1 muted purple bag, 4 muted coral bags.\nfaded teal bags contain 1 pale tan bag, 4 dark indigo bags, 1 posh olive bag.\ndotted orange bags contain 5 shiny brown bags, 3 striped plum bags, 3 plaid silver bags.\nplaid olive bags contain 1 posh white bag, 2 striped bronze bags, 2 dark gold bags, 3 plaid teal bags.\ndark lime bags contain 4 mirrored gray bags, 2 pale aqua bags.\nmirrored maroon bags contain 5 muted beige bags.\nshiny red bags contain 5 posh silver bags, 5 shiny blue bags.\ndrab magenta bags contain 4 muted plum bags, 4 light yellow bags.\nplaid purple bags contain no other bags.\ndrab indigo bags contain 1 dull blue bag, 3 wavy maroon bags, 5 pale gold bags, 3 pale crimson bags.\nvibrant white bags contain 1 dim salmon bag.\nmirrored teal bags contain 4 dotted chartreuse bags, 4 dim brown bags, 5 striped yellow bags.\nplaid gold bags contain 2 posh crimson bags, 5 muted green bags, 5 muted salmon bags, 1 pale plum bag.\nstriped indigo bags contain 2 muted beige bags, 4 mirrored fuchsia bags.\nbright purple bags contain 4 dim violet bags.\ndark salmon bags contain 2 clear silver bags, 5 wavy fuchsia bags, 5 bright salmon bags.\nmuted magenta bags contain 5 bright bronze bags, 1 dark red bag, 4 faded fuchsia bags.\ndrab olive bags contain 1 dim gold bag, 5 clear gold bags, 4 muted white bags.\nmirrored black bags contain 4 dim teal bags.\ndull bronze bags contain 3 dull white bags, 1 striped yellow bag, 1 striped crimson bag, 1 pale teal bag.\ndotted black bags contain 3 faded purple bags, 3 vibrant coral bags, 2 posh silver bags, 5 vibrant aqua bags.\ndrab aqua bags contain 1 striped lavender bag, 5 shiny lavender bags.\nshiny maroon bags contain 5 posh crimson bags, 4 drab blue bags, 1 pale black bag.\nfaded plum bags contain 2 posh tomato bags, 1 vibrant fuchsia bag, 2 faded black bags.\nwavy coral bags contain 5 shiny gold bags.\ndull brown bags contain 4 mirrored tan bags.\npale gray bags contain 5 dim maroon bags.\ndim tan bags contain 5 clear blue bags, 1 wavy bronze bag.\nplaid bronze bags contain 4 bright coral bags, 1 dotted crimson bag, 1 mirrored black bag."
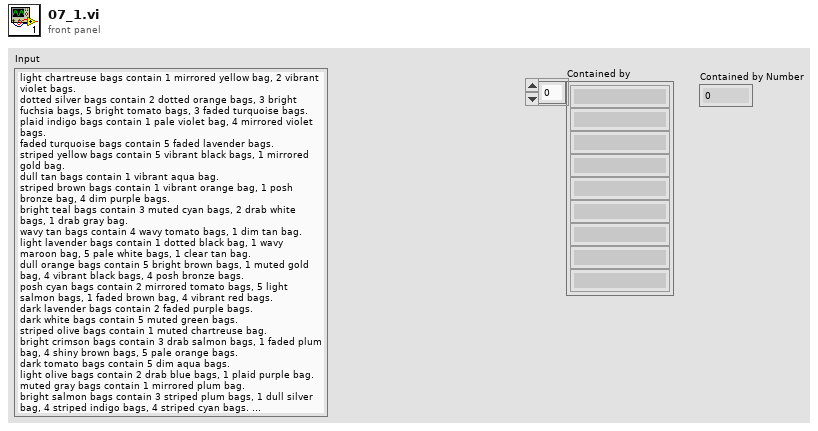
[diagram p1: front panel]
types:
  T1 = cluster{"Color":string, "Content":cluster{"Amount":i32, "Color":string}[]}
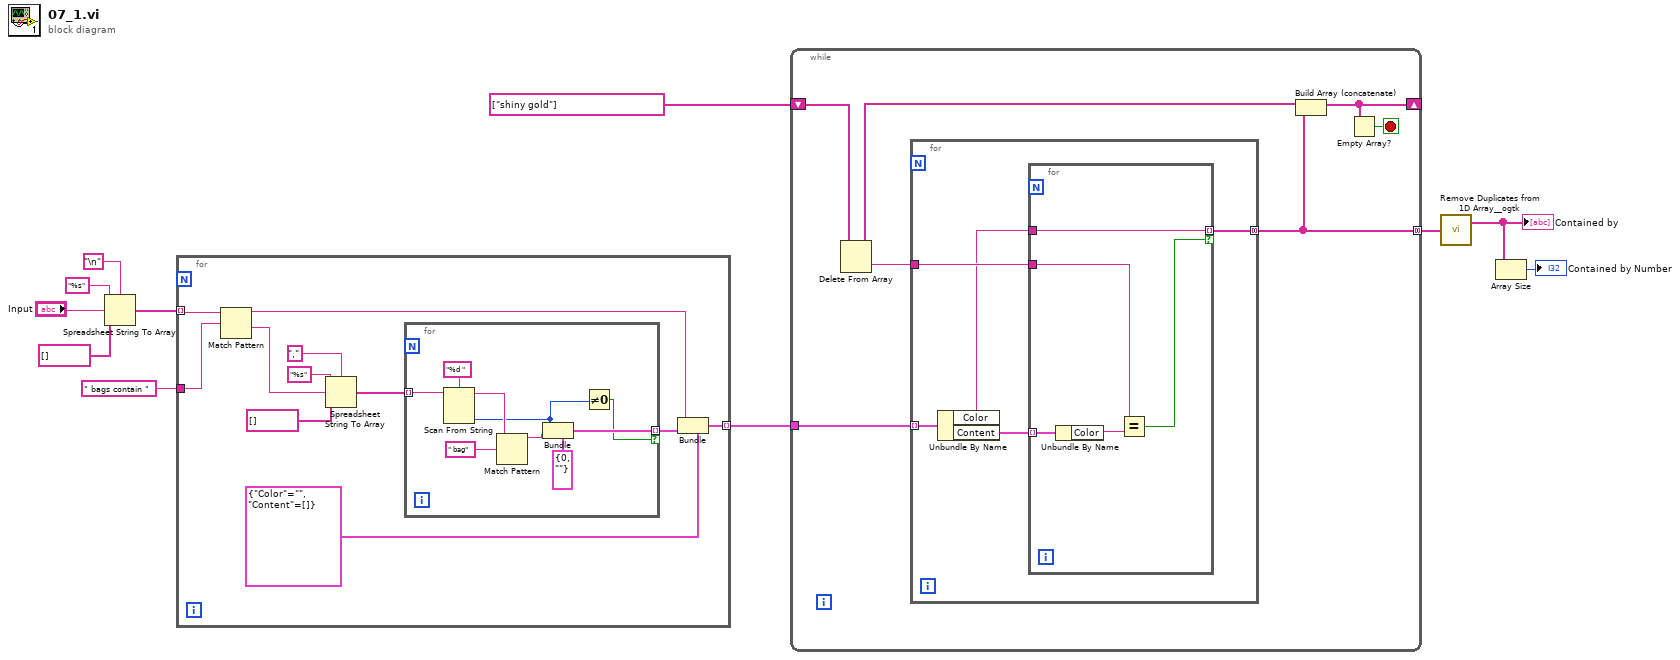
[diagram p0: block diagram]
diagram:
  n1 = Spreadsheet String To Array(delimiter (Tab)="\n", format string="%s", spreadsheet string="Input", array type (2D Dbl)=string[] []) -> (array=w7:string[])
  n2 = for {
    tunnel: w7 -> [w22] mode=indexing
    tunnel: " bags contain " -> [w21]
    tunnel: [w13] -> w4 mode=indexing
    n3 = Match Pattern(string=w22, regular expression=w21) -> (before substring=w14:string, after substring=w20:string)  [unwired: 1 in, 2 out]
    n4 = Spreadsheet String To Array(delimiter (Tab)=",", format string="%s", spreadsheet string=w20, array type (2D Dbl)=string[] []) -> (array=w16:string[])
    n5 = for {
      tunnel: w16 -> [w31] mode=indexing
      tunnel: [w27] -> w15 mode=indexing if=w23
      n6 = Scan From String(format string="%d ", input string=w31) -> (remaining string=w26:string, output 1=w24:i32)  [unwired: 3 in, 2 out]
      n7 = Match Pattern(string=w26, regular expression=" bag") -> (before substring=w28:string)  [unwired: 1 in, 3 out]
      n8 = Bundle(cluster=cluster{"Amount":i32, "Color":string} {"Amount"=0, "Color"=""}, "Amount"=w24, "Color"=w28) -> (w27:cluster{"Amount":i32, "Color":string})
      n9 = Not Equal To 0?(x=w24) -> (x != 0?=w23:bool)
    }
    n10 = Bundle(cluster=T1 {"Color"="", "Content"=[]}, "Color"=w14, "Content"=w15) -> (w13:T1)
  }
  n11 = while {
    shift-right: [w34] -> _
    shift-left: string[] ["shiny gold"] -> [w37]
    tunnel: w4 -> [w38]
    tunnel: [w32] -> w3 mode=concatenating
    stop <- w33 stop-if-true
    n12 = Delete From Array(array=w37) -> (deleted portion=w36:string, array with subset deleted=w35:string[])  [unwired: 2 in]
    n13 = for {
      tunnel: w38 -> [w43] mode=indexing
      tunnel: w36 -> [w41]
      tunnel: [w39] -> w32 mode=concatenating
      n14 = Unbundle By Name(w43) -> ("Color"=w40:string, "Content"=w42:cluster{"Amount":i32, "Color":string}[])
      n15 = for {
        tunnel: w42 -> [w48] mode=indexing
        tunnel: w41 -> [w46]
        tunnel: w40 -> [w45]
        tunnel: [w45] -> w39 mode=indexing if=w44
        n16 = Unbundle By Name(w48) -> ("Color"=w47:string)
        n17 = Equal?(x=w46, y=w47) -> (x = y?=w44:bool)
      }
    }
    n18 = Build Array (concatenate)(w35, w32) -> (w34:string[])
    n19 = Empty Array?(array=w34) -> (empty?=w33:bool)
  }
  n20 = call-poly <userlib>:"Remove Duplicates from 1D Array__ogtk.vi"("Input Array"=w3) -> ("Output Array"=w2:string[])  [unwired: 1 out]
  "Contained by" <- w2
  n21 = Array Size(array=w2) -> (size(s)=→"Contained by Number":i32)
